vi "Convert MAVLink Waypoints to Virtual.vi"(8 "Error In":errorcluster, 11 "Mavlink Waypoints":T1[](array[typedef])) -> (0 "Error Out":errorcluster)   [LabVIEW 2014]
uses:
  Controls/Mission Planning Controls/MAVLINK Mission Item.ctl
  Controls/MAVLINK Mav Frame.ctl
  Missions/Controls/Virtual Waypoint.ctl
  Missions/Controls/Waypoint Type.ctl
  Missions/FGVs/Virtual Waypoints/Methods/Clear All Virtual WP.vi
  Missions/FGVs/Virtual Waypoints/Methods/Get Virtual Waypoints.vi
  Missions/FGVs/Virtual Waypoints/Methods/Set Virtual Waypoints.vi
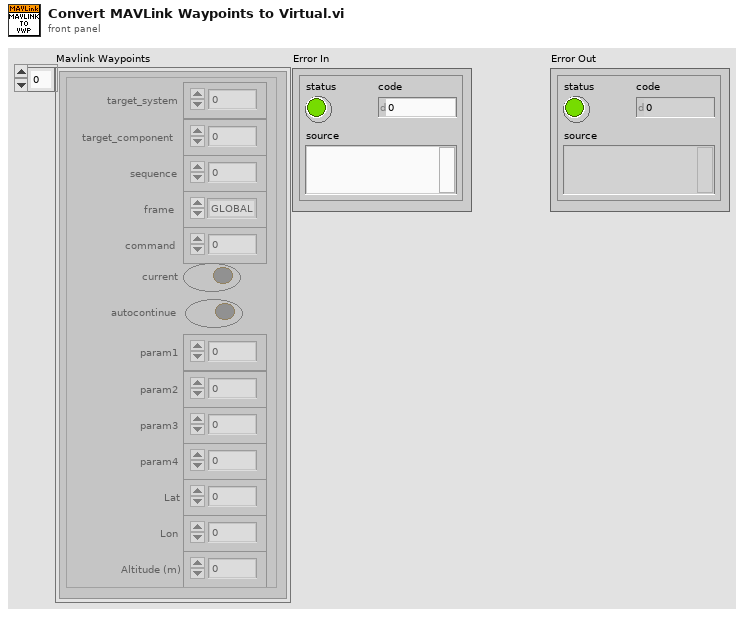
[diagram p1: front panel]
types:
  T1 = typedef "MAVLINK Mission Item.ctl" = cluster{"target_system":u8, "target_component":u8, "sequence":u16, "frame":T2, "command":u16, "current":bool, "autocontinue":bool, "param1":sgl, "param2":sgl, "param3":sgl, "param4":sgl, "Lat":sgl, "Lon":sgl, "Altitude (m)":sgl}
  T2 = typedef "MAVLINK Mav Frame.ctl" = enum8{"GLOBAL", "LOCAL NED", "MISSION", "GLOBAL RELATIVE ALT", "LOCAL ENU", "GLOBAL INT", "GLOBAL RELATIVE ALT INT", "LOCAL OFFSET NED", "BODY NED", "BODY OFFSET NED", "GLOBAL TERRAIN ALT", "GLOBAL TERRAIN ALT INT"}
  T3 = typedef "Virtual Waypoint.ctl" = cluster{"Waypoint Type":T4, "Lat":sgl, "Lon":sgl, "Altitude (m)":sgl, "Inspection Height (m)":sgl, "Circumnavigate Radius (m)":sgl, "Grid Waypoint?":bool, "Capture Photo":bool, "Speed (m/s)":sgl}
  T4 = typedef "Waypoint Type.ctl" = enum16{"PASS-THROUGH", "INSPECT", "CIRCUMNAVIGATE"}
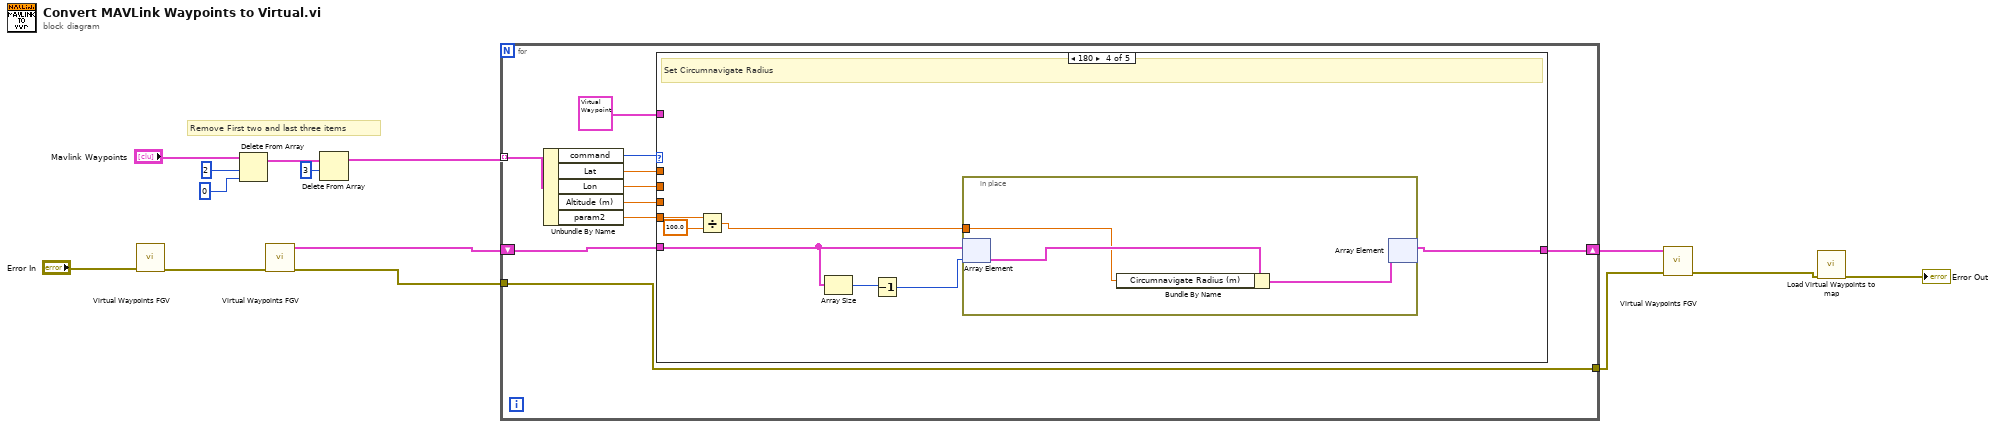
[diagram p0: block diagram]
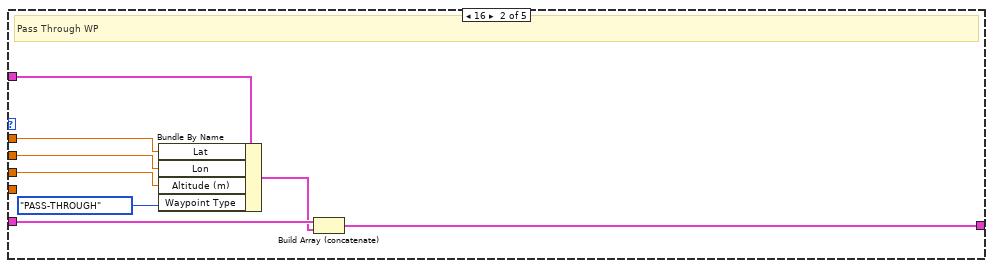
[diagram p3: hidden frame]
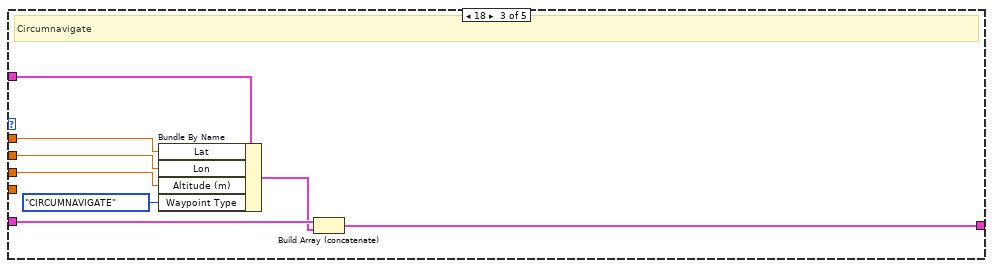
[diagram p4: hidden frame]
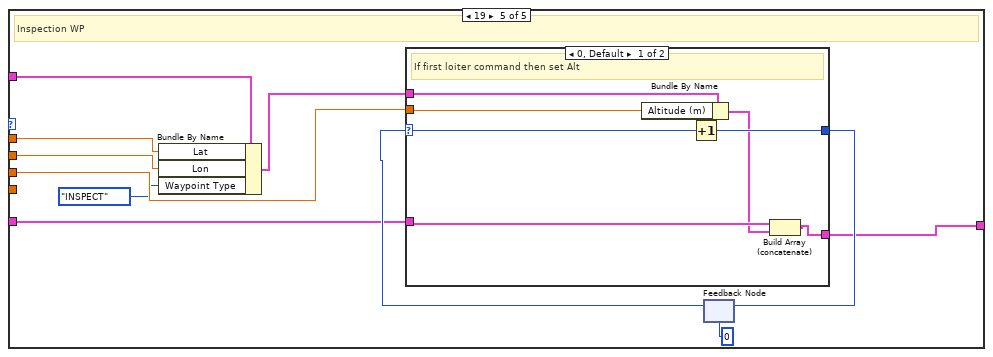
[diagram p5: hidden frame]
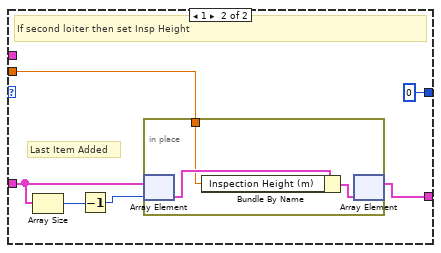
[diagram p6: hidden frame]
diagram:
  # "Remove First two and last three items"
  n1 = call-poly "Virtual Waypoints FGV.vi"("Error In"="Error In") -> ("Error Out"=w13:errorcluster)  [unwired: 10 in]
  n2 = Delete From Array(array="Mavlink Waypoints", length=2, index=0) -> (array with subset deleted=w7:T1[])  [unwired: 1 out]
  n3 = call-poly "Virtual Waypoints FGV.vi"("Error In"=w13) -> ("Error Out"=w11:errorcluster, "Virtual Waypoints Out"=w12:T3[])  [unwired: 9 in]
  n4 = Delete From Array(array=w7, length=3) -> (array with subset deleted=w5:T1[])  [unwired: 1 in, 1 out]
  n5 = for {
    tunnel: w5 -> [w24] mode=indexing
    shift-right: [w17] -> w4
    shift-left: w12 -> [w18]
    tunnel: w11 -> [w15]
    tunnel: [w15] -> w3
    n6 = Unbundle By Name(w24) -> ("command"=w23:u16, "Lat"=w19:sgl, "Lon"=w20:sgl, "Altitude (m)"=w21:sgl, "param2"=w16:sgl)
    n7 = case shown="180" w23 {
      tunnel: T3 {"Waypoint Type"=enum."PASS-THROUGH", "Lat"=0.0, "Lon"=0.0, "Altitude (m)"=0.0, "Inspection Height (m)"=0.0, "Circumnavigate Radius (m)"=0.0, "Grid Waypoint?"=FALSE, "Capture Photo"=FALSE, "Speed (m/s)"=0.0} ("Virtual Waypoints In") -> [_ w33 w41 _ w62]
      tunnel: w21 -> [_ w31 w40 _ w55]
      tunnel: w20 -> [_ w30 w39 _ w61]
      tunnel: w19 -> [_ w29 w38 _ w60]
      tunnel: w18 -> [w25 w28 w37 w48 w54]
      tunnel: [w25 w26 w35 w42 w53] -> w17
      tunnel: w16 -> [_ _ _ w45 _]
      frame 0, Default {
      }
      frame 16 {
        # "Pass Through WP"
        n8 = Bundle By Name(cluster=w33, "Lat"=w29, "Lon"=w30, "Altitude (m)"=w31, "Waypoint Type"=Waypoint_Type."PASS-THROUGH") -> (w27:T3)
        n9 = Build Array (concatenate)(w28, w27) -> (w26:T3[])
      }
      frame 18 {
        # "Circumnavigate"
        n10 = Bundle By Name(cluster=w41, "Lat"=w38, "Lon"=w39, "Altitude (m)"=w40, "Waypoint Type"=Waypoint_Type."CIRCUMNAVIGATE") -> (w36:T3)
        n11 = Build Array (concatenate)(w37, w36) -> (w35:T3[])
      }
      frame 180 {
        # "Set Circumnavigate Radius"
        n12 = Divide(x=w45, y=sgl 100.0) -> (x/y=w43:sgl)
        n13 = Array Size(array=w48) -> (size(s)=w47:i32)
        n14 = Decrement(x=w47) -> (x-1=w46:i32)
        n15 = in-place {
          in-place-border: w43 -> [w50]
          n16 = in-place-array #1(w48, w46) -> (w51:T3)
          n17 = Bundle By Name(cluster=w51, "Circumnavigate Radius (m)"=w50) -> (w49:T3)
          n18 = in-place-array #1(w49) -> (w42:T3[])  [unwired: 1 out]
        }
      }
      frame 19 {
        # "Inspection WP"
        n19 = Bundle By Name(cluster=w62, "Lat"=w60, "Lon"=w61, "Waypoint Type"=Waypoint_Type."INSPECT") -> (w56:T3)
        n20 = feedback #2(0) -> (w58:i32)
        n21 = case shown="0, Default" w58 {
          selector: w58 -> [w69 _]
          tunnel: [w68 0] -> w57
          tunnel: w56 -> [w67 _]
          tunnel: w55 -> [w66 w70]
          tunnel: w54 -> [w65 w74]
          tunnel: [w63 w71] -> w53
          frame 0, Default {
            # "If first loiter command then set Alt"
            n22 = Bundle By Name(cluster=w67, "Altitude (m)"=w66) -> (w64:T3)
            n23 = Increment(x=w69) -> (x+1=w68:i32)
            n24 = Build Array (concatenate)(w65, w64) -> (w63:T3[])
          }
          frame 1 {
            # "Last Item Added"
            # "If second loiter then set Insp Height"
            n25 = Array Size(array=w74) -> (size(s)=w73:i32)
            n26 = Decrement(x=w73) -> (x-1=w72:i32)
            n27 = in-place {
              in-place-border: w70 -> [w76]
              n28 = in-place-array #3(w74, w72) -> (w78:T3)
              n29 = Bundle By Name(cluster=w78, "Inspection Height (m)"=w76) -> (w77:T3)
              n30 = in-place-array #3(w77) -> (w71:T3[])  [unwired: 1 out]
            }
          }
        }
        n31 = feedback-in #2(w57) -> ()
      }
    }
  }
  n32 = call-poly "Virtual Waypoints FGV.vi"("Error In"=w3, "Virtual Waypoints In"=w4) -> ("Error Out"=w2:errorcluster)  [unwired: 9 in]
  n33 = call "Load Virtual Waypoints to map.vi"("Error In"=w2) -> ("Error Out"=→"Error Out":errorcluster)  [unwired: 10 in]
